vi "FTW-Test-Actor-InboxConfiguration.vi"() -> (0 "Test Result":errorcluster)   [LabVIEW 2015]
uses:
  src/socket/inbox/core/FTW-Inbox-Core-RoutingRule.ctl
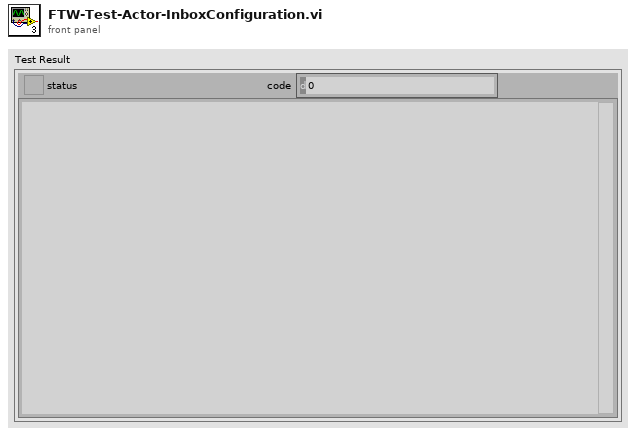
[diagram p1: front panel]
types:
  T1 = typedef "FTW-Inbox-Core-RoutingRule.ctl" = cluster{"Pattern":string, "BusyTimeout":i32, "SendTimeout":i32, "Accept":bool, "Reject":bool, "ReplyWithIdentity":bool, "ReplyWithStatus":bool, "ReplyWithTimestamp":bool, "ReplyWithRelativeTimer":bool, "AutoReply":bool}
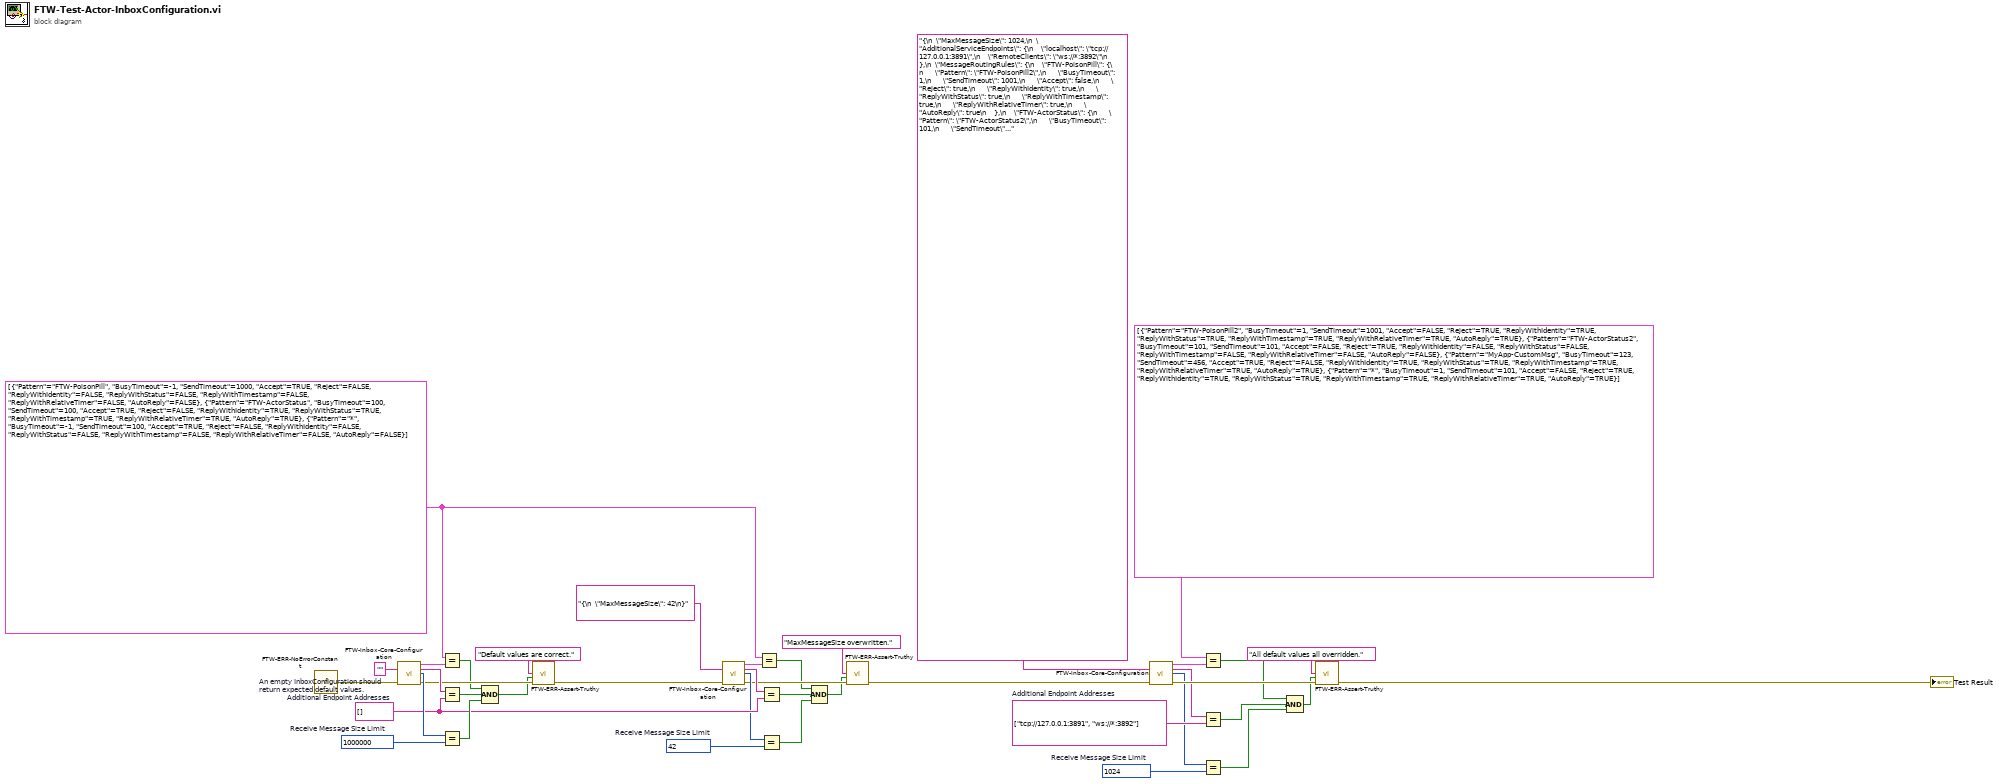
[diagram p0: block diagram]
diagram:
  w9 = 42  # Receive Message Size Limit
  w21 = 1024  # Receive Message Size Limit
  w20 = string[] ["tcp://127.0.0.1:3891", "ws://*:3892"]  # Additional Endpoint Addresses
  w29 = 1000000  # Receive Message Size Limit
  w11 = string[] []  # Additional Endpoint Addresses
  w13 = T1[] [{"Pattern"="FTW-PoisonPill", "BusyTimeout"=-1, "SendTimeout"=1000, "Accept"=TRUE, "Reject"=FALSE, "ReplyWithIdentity"=FALSE, "ReplyWithStatus"=FALSE, "ReplyWithTimestamp"=FALSE, "ReplyWithRelativeTimer"=FALSE, "AutoReply"=FALSE}, {"Pattern"="FTW-ActorStatus", "BusyTimeout"=100, "SendTimeout"=100, "Accept"=TRUE, "Reject"=FALSE, "ReplyWithIdentity"=TRUE, "ReplyWithStatus"=TRUE, "ReplyWithTimestamp"=TRUE, "ReplyWithRelativeTimer"=TRUE, "AutoReply"=TRUE}, {"Pattern"="*", "BusyTimeout"=-1, "SendTimeout"=100, "Accept"=TRUE, "Reject"=FALSE, "ReplyWithIdentity"=FALSE, "ReplyWithStatus"=FALSE, "ReplyWithTimestamp"=FALSE, "ReplyWithRelativeTimer"=FALSE, "AutoReply"=FALSE}] ("Message Routing Rules")
  w37 = ""  # An empty InboxConfiguration should return expected default values.
  n1 = call "FTW-ERR-NoErrorConstant.vi"() -> ("no error"=w38:errorcluster)
  n2 = call "FTW-Inbox-Core-Configuration.vi"("Inbox Configuration"=w37, "error in"=w38) -> ("Message Routing Rules"=w36:T1[], "Additional Endpoint Addresses"=w35:string[], "Receive Message Size Limit"=w34:i32, "error out"=w33:errorcluster)  [unwired: 10 in]
  n3 = Equal?(x=w13, y=w36) -> (x = y?=w32:bool)
  n4 = Equal?(x=w35, y=w11) -> (x = y?=w31:bool)
  n5 = Equal?(x=w34, y=w29) -> (x = y?=w30:bool)
  n6 = Compound Arithmetic op=AND(w32, w31, w30) -> (w28:bool)
  n7 = call "FTW-ERR-Assert-Truthy.vi"("Assertion"="Default values are correct.", "Assertion holds true?"=w28, "error in"=w33) -> ("error out"=w14:errorcluster)  [unwired: 12 in]
  n8 = call "FTW-Inbox-Core-Configuration.vi"("Inbox Configuration"="{\n  \"MaxMessageSize\": 42\n}", "error in"=w14) -> ("Message Routing Rules"=w12:T1[], "Additional Endpoint Addresses"=w10:string[], "Receive Message Size Limit"=w8:i32, "error out"=w6:errorcluster)  [unwired: 10 in]
  n9 = Equal?(x=w13, y=w12) -> (x = y?=w3:bool)
  n10 = Equal?(x=w10, y=w11) -> (x = y?=w4:bool)
  n11 = Equal?(x=w8, y=w9) -> (x = y?=w2:bool)
  n12 = Compound Arithmetic op=AND(w3, w4, w2) -> (w1:bool)
  n13 = call "FTW-ERR-Assert-Truthy.vi"("Assertion"="MaxMessageSize overwritten.", "Assertion holds true?"=w1, "error in"=w6) -> ("error out"=w5:errorcluster)  [unwired: 12 in]
  n14 = call "FTW-Inbox-Core-Configuration.vi"("Inbox Configuration"="{\n  \"MaxMessageSize\": 1024,\n  \"AdditionalServiceEndpoints\": {\n    \"localhost\": \"tcp://127.0.0.1:3891\",\n    \"RemoteClients\": \"ws://*:3892\"\n  },\n  \"MessageRoutingRules\": {\n    \"FTW-PoisonPill\": {\n      \"Pattern\": \"FTW-PoisonPill2\",\n      \"BusyTimeout\": 1,\n      \"SendTimeout\": 1001,\n      \"Accept\": false,\n      \"Reject\": true,\n      \"ReplyWithIdentity\": true,\n      \"ReplyWithStatus\": true,\n      \"ReplyWithTimestamp\": true,\n      \"ReplyWithRelativeTimer\": true,\n      \"AutoReply\": true\n    },\n    \"FTW-ActorStatus\": {\n      \"Pattern\": \"FTW-ActorStatus2\",\n      \"BusyTimeout\": 101,\n      \"SendTimeout\": 101,\n      \"Accept\": false,\n      \"Reject\": true,\n      \"ReplyWithIdentity\": false,\n      \"ReplyWithStatus\": false,\n      \"ReplyWithTimestamp\": false,\n      \"ReplyWithRelativeTimer\": false,\n      \"AutoReply\": false\n    },\n    \"Custom\": {\n      \"Pattern\": \"MyApp-CustomMsg\",\n      \"BusyTimeout\": 123,\n      \"SendTimeout\": 456,\n      \"Accept\": true,\n      \"Reject\": false,\n      \"ReplyWithIdentity\": true,\n      \"ReplyWithStatus\": true,\n      \"ReplyWithTimestamp\": true,\n      \"ReplyWithRelativeTimer\": true,\n      \"AutoReply\": true\n    },\n    \"Default\": {\n      \"Pattern\": \"*\",\n      \"BusyTimeout\": 1,\n      \"SendTimeout\": 101,\n      \"Accept\": false,\n      \"Reject\": true,\n      \"ReplyWithIdentity\": true,\n      \"ReplyWithStatus\": true,\n      \"ReplyWithTimestamp\": true,\n      \"ReplyWithRelativeTimer\": true,\n      \"AutoReply\": true\n    }\n  }\n}", "error in"=w5) -> ("Message Routing Rules"=w25:T1[], "Additional Endpoint Addresses"=w18:string[], "Receive Message Size Limit"=w19:i32, "error out"=w26:errorcluster)  [unwired: 10 in]
  n15 = Equal?(x=T1[] [{"Pattern"="FTW-PoisonPill2", "BusyTimeout"=1, "SendTimeout"=1001, "Accept"=FALSE, "Reject"=TRUE, "ReplyWithIdentity"=TRUE, "ReplyWithStatus"=TRUE, "ReplyWithTimestamp"=TRUE, "ReplyWithRelativeTimer"=TRUE, "AutoReply"=TRUE}, {"Pattern"="FTW-ActorStatus2", "BusyTimeout"=101, "SendTimeout"=101, "Accept"=FALSE, "Reject"=TRUE, "ReplyWithIdentity"=FALSE, "ReplyWithStatus"=FALSE, "ReplyWithTimestamp"=FALSE, "ReplyWithRelativeTimer"=FALSE, "AutoReply"=FALSE}, {"Pattern"="MyApp-CustomMsg", "BusyTimeout"=123, "SendTimeout"=456, "Accept"=TRUE, "Reject"=FALSE, "ReplyWithIdentity"=TRUE, "ReplyWithStatus"=TRUE, "ReplyWithTimestamp"=TRUE, "ReplyWithRelativeTimer"=TRUE, "AutoReply"=TRUE}, {"Pattern"="*", "BusyTimeout"=1, "SendTimeout"=101, "Accept"=FALSE, "Reject"=TRUE, "ReplyWithIdentity"=TRUE, "ReplyWithStatus"=TRUE, "ReplyWithTimestamp"=TRUE, "ReplyWithRelativeTimer"=TRUE, "AutoReply"=TRUE}] ("Message Routing Rules"), y=w25) -> (x = y?=w23:bool)
  n16 = Equal?(x=w18, y=w20) -> (x = y?=w17:bool)
  n17 = Equal?(x=w19, y=w21) -> (x = y?=w16:bool)
  n18 = Compound Arithmetic op=AND(w23, w17, w16) -> (w22:bool)
  n19 = call "FTW-ERR-Assert-Truthy.vi"("Assertion"="All default values all overridden.", "Assertion holds true?"=w22, "error in"=w26) -> ("error out"=→"Test Result":errorcluster)  [unwired: 12 in]
